vi "Select Data.vi"(7 "WHERE Statement":string, 8 "error in (no error)":errorcluster, 9 "Columns":string[](array[string]), 10 "Table":string, 11 "ADODB in":refnum<class "ADODB.lvclass">) -> (0 "error out":errorcluster, 2 "Data":string[][](table), 3 "ADODB out":refnum<class "ADODB.lvclass">)   [LabVIEW 2020, in "ADODB.lvclass"]
uses:
  ADODB.lvclass
  ADODB.lvclass/ADODB.ctl
  <vilib>/addons/database/_DB Variant To Data/Database Variant To Data.xnode
  <vilib>/addons/database/NI_Database_API.lvlib
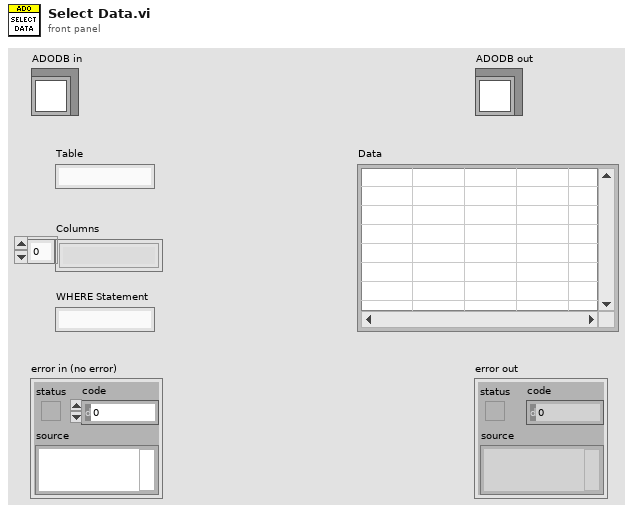
[diagram p1: front panel]
types:
  T1 = typedef "NI_Database_API.lvlib/Conn ObjectReference.ctl" = refnum<k1>
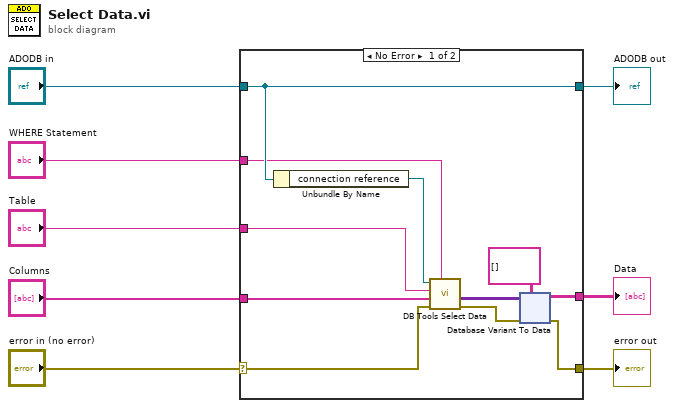
[diagram p0: block diagram]
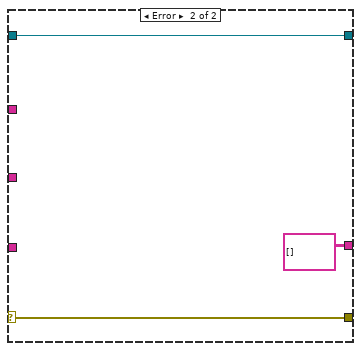
[diagram p2: hidden frame]
diagram:
  n1 = case shown="No Error" "error in (no error)" {
    selector: "error in (no error)" -> [w14 w66]
    tunnel: [w11 w66] -> w7
    tunnel: "ADODB in" -> [w19 w65]
    tunnel: [w19 w65] -> w5
    tunnel: "Columns" -> [w15 _]
    tunnel: "Table" -> [w16 _]
    tunnel: "WHERE Statement" -> [w17 _]
    tunnel: [w9 string[][] [] ("data")] -> w1
    frame No Error {
      n2 = Unbundle By Name(w19) -> ("connection reference"=w18:T1)
      n3 = call <vilib>:"DB Tools Select Data.vi"("condition"=w17, "error in (no error)"=w14, "columns"=w15, "table"=w16, "connection reference"=w18) -> ("error out"=w12:errorcluster, "data"=w13:variant[][])  [unwired: 1 in, 1 out]
      n4 = xnode "Database Variant To Data"("database variant"=w13, "error in (no error)"=w12, "type"=string[][] []) -> ("data"=w9:string[][], "error out"=w11:errorcluster)
    }
    frame Error {
    }
  }
  "error out" <- w7
  "ADODB out" <- w5
  "Data" <- w1
